vi "FG-Image-height.vi"(8 "error in":errorcluster, 10 "Config file string in":string, 11 "Config. params. ref. in":refnum<data-value>) -> (0 "error IO":errorcluster, 1 "Number of replacements":i32, 2 "Config file string":string, 3 "Config. params. ref.":refnum<data-value>)   [LabVIEW 2013, in "CameraVision.lvlib" / "CV-Configuration.lvclass"]
uses:
  CV-Configuration.lvclass
  CV-Configuration.lvclass/CV-Configuration.ctl
  Hardware/Camera/Camera.lvclass/Camera.ctl
  Read ROI height.vi
  Read Framegrabber DLL file.vi
  Read BoardHandle.vi
  Read Camport array.vi
  Read Camera array.vi
  Hardware/Camera/Camera.lvclass
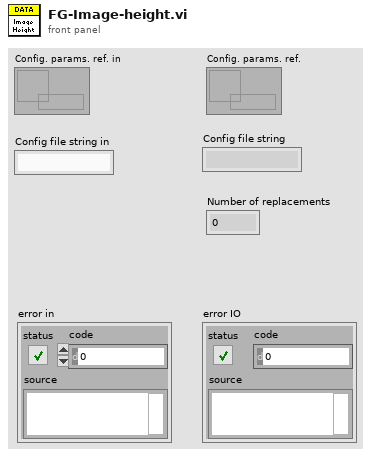
[diagram p1: front panel]
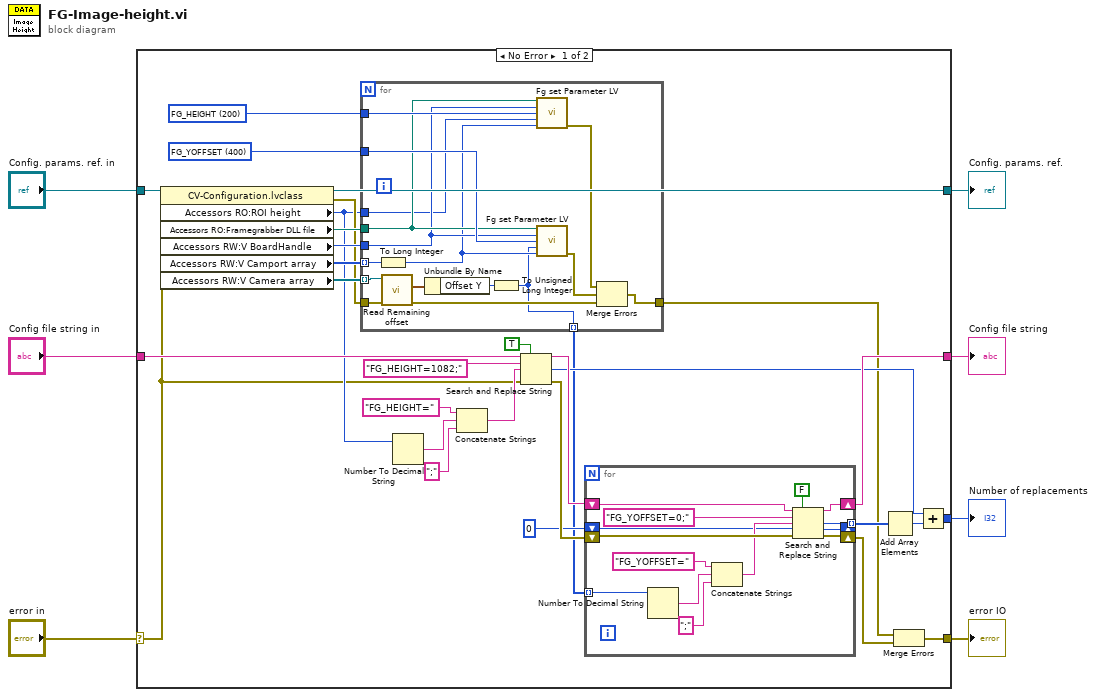
[diagram p0: block diagram]
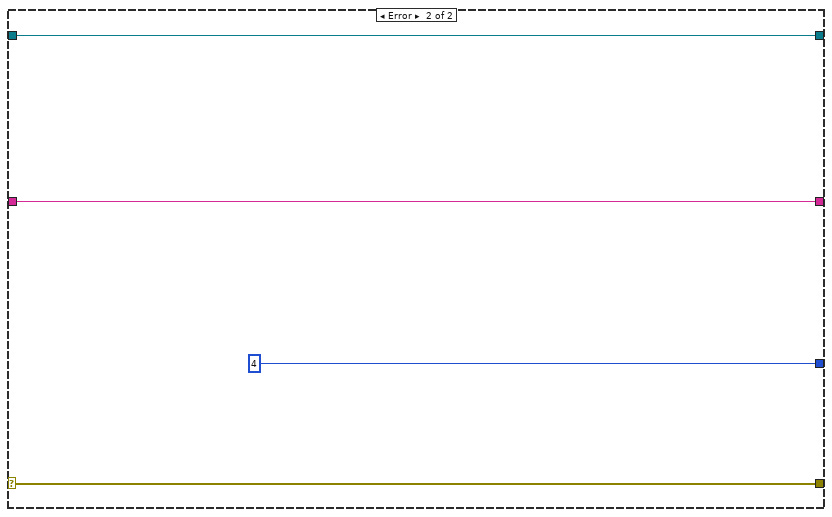
[diagram p2: hidden frame]
diagram:
  n1 = case shown="No Error" "error in" {
    selector: "error in" -> [w8 w70]
    tunnel: [w37 4] -> w4
    tunnel: [w12 w70] -> w3
    tunnel: [w35 w69] -> w5
    tunnel: "Config file string in" -> [w34 w69]
    tunnel: "Config. params. ref. in" -> [w15 w68]
    tunnel: [w14 w68] -> w1
    frame No Error {
      w19 = 200 items=["FG_WIDTH"=100, "FG_HEIGHT"=200, "FG_FORMAT"=700, "FG_XOFFSET"=300, "FG_YOFFSET"=400, "FG_FRAMESPERSEC"=90, "FG_EXPOSURE"=10020, "FG_TRIGGERMODE"=8100, "FG_TRIGGERINSRC"=8110, "FG_CAMERA_LINK_CAMTYP"=11011, "FG_USEDVAL"=5025, "FG_SENSORREADOUT"=5050, "FG_STROBEPULSEDELAY"=8700, "FG_FLASH_POLARITY"=24060, "FG_EXSYNCINVERT"=8200, "FG_EXSYNCPOLARITY"=8420, "FG_EXSYNCDELAY"=8400, "FG_FLASHON"=8600, "FG_EXSYNCON"=8300, "FG_TRIGGERINPOLARITY"=8116, "FG_KNEE_LUT_FILE"=12110, "FG_KNEE_LUT_OFFSET"=12102, "FG_KNEE_LUT_SCALE"=12101, "FG_KNEE_LUT_GAMMA"=12103, "FG_KNEE_LUT_INVERT"=12104, "FG_CCSEL0"=14001, "FG_CCSEL1"=14002, "FG_CCSEL2"=14003, "FG_CCSEL3"=14004, "FG_DIGIO_OUTPUT"=14020, "FG_IMG_SELECT_PERIOD"=25110, "FG_IMG_SELECT"=25111, "FG_PORT"=3000, "FG_GLOBAL_ACCESS"=24110, "FG_TIMEOUT"=600] ("Ring")
      w20 = 400 items=["FG_WIDTH"=100, "FG_HEIGHT"=200, "FG_FORMAT"=700, "FG_XOFFSET"=300, "FG_YOFFSET"=400, "FG_FRAMESPERSEC"=90, "FG_EXPOSURE"=10020, "FG_TRIGGERMODE"=8100, "FG_TRIGGERINSRC"=8110, "FG_CAMERA_LINK_CAMTYP"=11011, "FG_USEDVAL"=5025, "FG_SENSORREADOUT"=5050, "FG_STROBEPULSEDELAY"=8700, "FG_FLASH_POLARITY"=24060, "FG_EXSYNCINVERT"=8200, "FG_EXSYNCPOLARITY"=8420, "FG_EXSYNCDELAY"=8400, "FG_FLASHON"=8600, "FG_EXSYNCON"=8300, "FG_TRIGGERINPOLARITY"=8116, "FG_KNEE_LUT_FILE"=12110, "FG_KNEE_LUT_OFFSET"=12102, "FG_KNEE_LUT_SCALE"=12101, "FG_KNEE_LUT_GAMMA"=12103, "FG_KNEE_LUT_INVERT"=12104, "FG_CCSEL0"=14001, "FG_CCSEL1"=14002, "FG_CCSEL2"=14003, "FG_CCSEL3"=14004, "FG_DIGIO_OUTPUT"=14020, "FG_IMG_SELECT_PERIOD"=25110, "FG_IMG_SELECT"=25111, "FG_PORT"=3000, "FG_GLOBAL_ACCESS"=24110, "FG_TIMEOUT"=600] ("Ring")
      n2 = property class="CV-Configuration.lvclass"(reference=w15, error in=w8) -> (reference out=w14:refnum<data-value>, error out=w16:errorcluster, "Accessors RO:ROI height"=w10:u32, "Accessors RO:Framegrabber DLL file"=w17:path, "Accessors RW:V BoardHandle"=w21:u64, "Accessors RW:V Camport array"=w18:u32[], "Accessors RW:V Camera array"=w22:refnum<class "Camera.lvclass">[])
      n3 = for {
        tunnel: w22 -> [w53] mode=indexing
        tunnel: w17 -> [w47]
        tunnel: w21 -> [w46]
        tunnel: w20 -> [w49]
        tunnel: w19 -> [w48]
        tunnel: w18 -> [w45] mode=indexing
        tunnel: w10 -> [w43]
        tunnel: [w38] -> w9 mode=indexing
        tunnel: w16 -> [w52]
        tunnel: [w41] -> w11
        n4 = To Long Integer(number=w45) -> (32bit integer=w44:i32)
        n5 = call "Read Remaining offset.vi"("error in (no error)"=w52, "Camera in"=w53) -> ("error out"=w51:errorcluster, "Remaining offset"=w50:cluster{"Offset X":i32, "Offset Y":i32})  [unwired: 7 in, 1 out]
        n6 = Unbundle By Name(w50) -> ("Offset Y"=w42:i32)
        n7 = To Unsigned Long Integer(number=w42) -> (unsigned 32bit integer=w38:u32)
        n8 = call <userlib>:"Fg set Parameter LV.vi"("dll path in"=w47, "FgAddr"=w46, "Parameter"=w48, "Value"=w43, "CamPort"=w44) -> ("error out"=w39:errorcluster)  [unwired: 8 in, 2 out]
        n9 = call <userlib>:"Fg set Parameter LV.vi"("dll path in"=w47, "FgAddr"=w46, "Parameter"=w49, "Value"=w38, "CamPort"=w44) -> ("error out"=w40:errorcluster)  [unwired: 8 in, 2 out]
        n10 = Merge Errors(w39, w40, w51) -> (w41:errorcluster)
      }
      n11 = Number To Decimal String(number=w10) -> (decimal integer string=w31:string)  [unwired: 1 in]
      n12 = Concatenate Strings("FG_HEIGHT=" ("string"), w31, ";" ("string")) -> (w29:string)
      n13 = Search and Replace String(replace all?=TRUE, input string=w34, search string="FG_HEIGHT=1082;", replace string=w29, error in=w8) -> (result string=w27:string, number of replacements=w26:i32, error out=w28:errorcluster)  [unwired: 3 in, 1 out]
      n14 = for {
        tunnel: [w60] -> w23 mode=indexing
        tunnel: w9 -> [w54] mode=indexing
        shift-right: [w66] -> w35
        shift-left: w27 -> [w61]
        shift-right: [w56] -> _
        shift-left: 0 ("offset (0)") -> [w57]
        shift-right: [w67] -> w36
        shift-left: w28 -> [w62]
        n15 = Number To Decimal String(number=w54) -> (decimal integer string=w64:string)  [unwired: 1 in]
        n16 = Concatenate Strings("FG_YOFFSET=" ("string"), w64, ";" ("string")) -> (w58:string)
        n17 = Search and Replace String(replace all?=FALSE ("replace all? (F)"), input string=w61, search string="FG_YOFFSET=0;", replace string=w58, offset=w57, error in=w62) -> (result string=w66:string, number of replacements=w60:i32, offset past replacement=w56:i32, error out=w67:errorcluster)  [unwired: 2 in]
      }
      n18 = Add Array Elements(numeric array=w23) -> (sum=w24:i32)
      n19 = Merge Errors(w11, w36) -> (w12:errorcluster)
      n20 = Add(x=w26, y=w24) -> (x+y=w37:i32)
    }
    frame Error {
    }
  }
  "Number of replacements" <- w4
  "error IO" <- w3
  "Config file string" <- w5
  "Config. params. ref." <- w1
